vi "AvoidOwnGoal.vi"(0 "DefendAreaTactic in":refnum<class "DefendAreaTactic.lvclass">, 1 "Field":refnum<class "Field.lvclass">, 3 "Robot":refnum<class "Robot.lvclass">, 5 "error in (no error)":errorcluster) -> (14 "DefendAreaTactic out":refnum<class "DefendAreaTactic.lvclass">, 16 "Is shooting to our goal?":bool, 19 "error out":errorcluster)   [LabVIEW 2024, in "DefendAreaTactic.lvclass"]
uses:
  DefendAreaTactic.lvclass
  Robot_class/Robot.lvclass
  C:/Users/ROBOIME2/Documents/SSL ROBOIME/SSL_AI/Object_class/Object.lvclass
  Field_class/Field.lvclass
  Object_class/Object.lvclass/Object.ctl
  Robot_class/Robot.lvclass/Robot.ctl
  Object_class/Read x.vi
  Object_class/Read y.vi
  Robot_class/Read orientation.vi
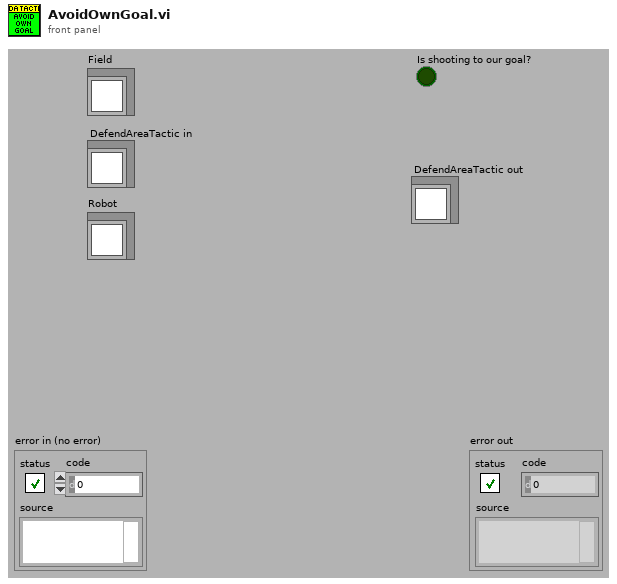
[diagram p1: front panel]
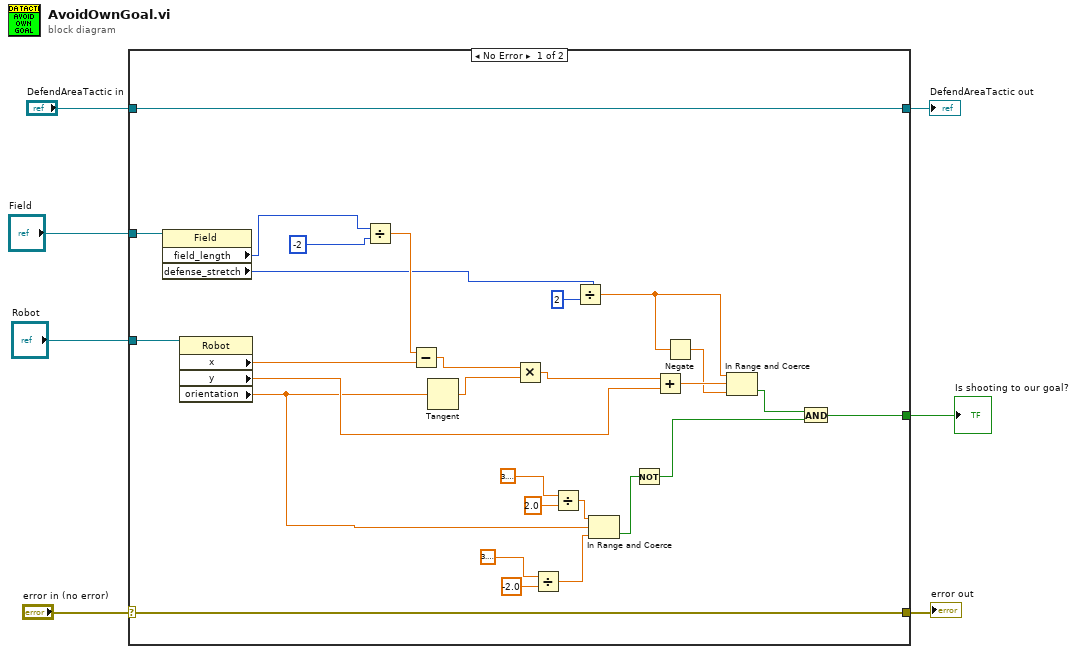
[diagram p0: block diagram]
diagram:
  n1 = case shown="No Error" "error in (no error)" {
    selector: "error in (no error)" -> [w34 w37]
    tunnel: [w34 w37] -> w6
    tunnel: [w35 w36] -> w4
    tunnel: "DefendAreaTactic in" -> [w35 w36]
    tunnel: "Robot" -> [w33 _]
    tunnel: "Field" -> [w25 _]
    tunnel: [w12 _] -> w1
    frame No Error {
      n2 = property class="Field"(reference=w25) -> ("field_length"=w24:i32, "defense_stretch"=w23:i32)  [unwired: 1 in, 2 out]
      n3 = property class="Robot"(reference=w33) -> ("x"=w32:dbl, "y"=w27:dbl, "orientation"=w8:dbl)  [unwired: 1 in, 2 out]
      n4 = Divide(x=w24, y=-2) -> (x/y=w31:dbl)
      n5 = Subtract(x=w31, y=w32) -> (x-y=w30:dbl)
      n6 = Tangent(1:w8) -> (0:w29:dbl)
      n7 = Multiply(x=w30, y=w29) -> (x*y=w28:dbl)
      n8 = Divide(x=3.141592653589793, y=-2.0) -> (x/y=w14:dbl)
      n9 = Divide(x=3.141592653589793, y=2.0) -> (x/y=w13:dbl)
      n10 = Divide(x=w23, y=2) -> (x/y=w21:dbl)
      n11 = In Range and Coerce(upper limit=w13, x=w8, lower limit=w14) -> (In Range?=w9:bool)  [unwired: 1 out]
      n12 = Not(x=w9) -> (.not. x?=w10:bool)
      n13 = Add(x=w28, y=w27) -> (x+y=w26:dbl)
      n14 = Negate(x=w21) -> (-x=w20:dbl)
      n15 = In Range and Coerce(upper limit=w21, x=w26, lower limit=w20) -> (In Range?=w19:bool)  [unwired: 1 out]
      n16 = And(x=w19, y=w10) -> (x .and. y?=w12:bool)
    }
    frame Error {
    }
  }
  "error out" <- w6
  "DefendAreaTactic out" <- w4
  "Is shooting to our goal?" <- w1
